vi "Update Controls State.vi"(6 "Controls Need Update In":bool, 7 "Controlst In":refnum<vi>, 8 "Error In (no Error) In":errorcluster, 9 "DigNum Refnum In":refnum<vi>, 10 "Str Refnum In":refnum<vi>, 11 "Display State In":T1={"Show Axes"=FALSE, "Show Y=0"=FALSE, "Controls"={"Type"=enum."Sine", "Periods"=0.0, "Points"=0, "Offset"=0.0, "Amplitdue"=0.0, "Phase"=0.0, "func"=""}, "Show Current Location"=FALSE, "Current Location"=0, "dt"=0.0, "t0"=timestamp(0 s since 1904-01-01), "Format and Units"="%_3p"} caption="State") -> (0 "Error Out":errorcluster, 3 "Display State Out":T1={"Show Axes"=FALSE, "Show Y=0"=FALSE, "Controls"={"Type"=enum."Sine", "Periods"=0.0, "Points"=0, "Offset"=0.0, "Amplitdue"=0.0, "Phase"=0.0, "func"=""}, "Show Current Location"=FALSE, "Current Location"=0, "dt"=0.0, "t0"=timestamp(0 s since 1904-01-01), "Format and Units"="%_3p"} caption="State")   [LabVIEW 2012, in "Waveform Control.xctl"]
doc: "Updates the function generator controls from the state"
uses:
  Waveform Control.xctl
  Controls/Waveform State.ctl
  FP Controls.ctl
  Function Types.ctl
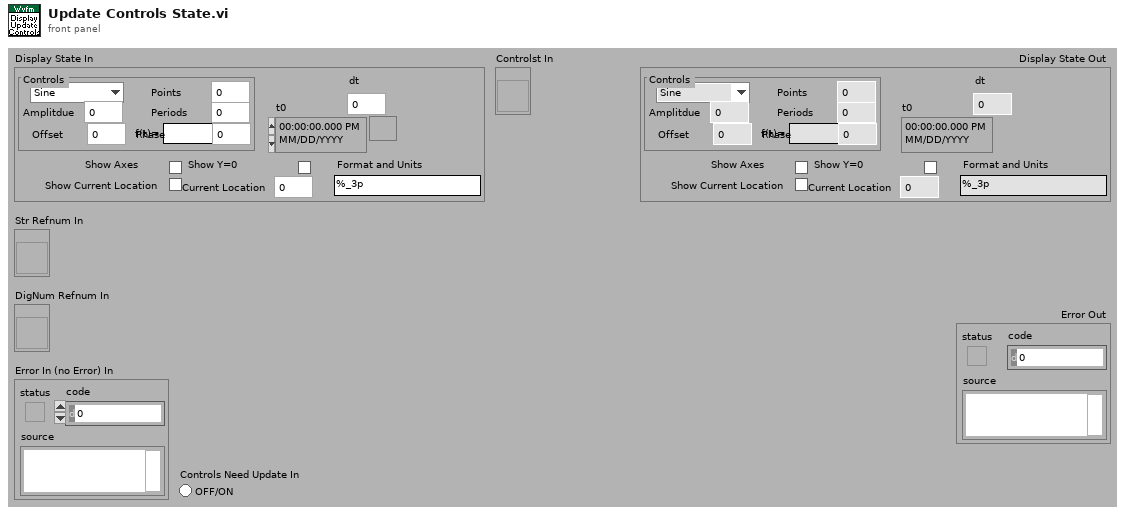
[diagram p1: front panel]
types:
  T1 = typedef "Waveform Control.xctl/Waveform State.ctl" = cluster{"Show Axes":bool, "Show Y=0":bool, "Controls":T2, "Show Current Location":bool, "Current Location":i32, "dt":dbl, "t0":timestamp, "Format and Units":string}
  T2 = typedef "Waveform Control.xctl/FP Controls.ctl" = cluster{"Type":T3, "Periods":dbl, "Points":i32, "Offset":dbl, "Amplitdue":dbl, "Phase":dbl, "func":string}
  T3 = typedef "Waveform Control.xctl/Function Types.ctl" = enum16{"Level", "Sine", "Triangle", "Ramp", "Saw Tooth", "Square", "Function"}
  T4 = cluster{"Type":T3, "Periods":dbl, "Points":i32, "Offset":dbl, "Amplitdue":dbl, "Starting Phase":dbl, "func":string}
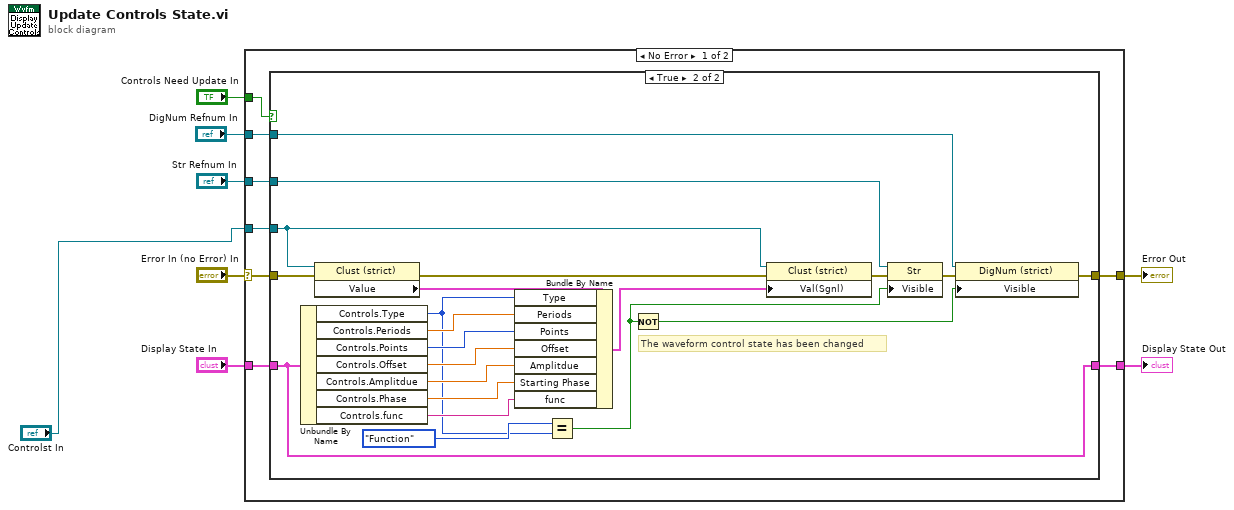
[diagram p0: block diagram]
diagram:
  n1 = case shown="No Error" "Error In (no Error) In" {
    selector: "Error In (no Error) In" -> [w10 w40]
    tunnel: [w16 w40] -> w8
    tunnel: "Display State In" -> [w15 _]
    tunnel: "Controlst In" -> [w14 _]
    tunnel: "Str Refnum In" -> [w13 _]
    tunnel: "DigNum Refnum In" -> [w12 _]
    tunnel: "Controls Need Update In" -> [w9 _]
    tunnel: [w11 _] -> w2
    frame No Error {
      n2 = case shown="True" w9 {
        tunnel: [w17 w39] -> w16
        tunnel: w15 -> [w18 w20]
        tunnel: w14 -> [_ w38]
        tunnel: w13 -> [_ w37]
        tunnel: w12 -> [_ w36]
        tunnel: [w18 w20] -> w11
        tunnel: w10 -> [w17 w19]
        frame False {
        }
        frame True {
          # "The waveform control state has been changed"
          n3 = Unbundle By Name(w20) -> ("Controls.Type"=w21:T3, "Controls.Periods"=w30:dbl, "Controls.Points"=w29:i32, "Controls.Offset"=w28:dbl, "Controls.Amplitdue"=w27:dbl, "Controls.Phase"=w26:dbl, "Controls.func"=w25:string)
          n4 = property on="Property Node" class="Clust (strict)"(reference=w38, error in=w19) -> (error out=w22:errorcluster, "Value"=w31:T4)  [unwired: 1 out]
          n5 = Bundle By Name(cluster=w31, "Type"=w21, "Periods"=w30, "Points"=w29, "Offset"=w28, "Amplitdue"=w27, "Starting Phase"=w26, "func"=w25) -> (w24:T4)
          n6 = Equal?(x=Function_Types."Function" ("Type"), y=w21) -> (x = y?=w34:bool)
          n7 = Not(x=w34) -> (.not. x?=w33:bool)
          n8 = property on="Property Node" class="Clust (strict)"(reference=w38, error in=w22, "Val(Sgnl)"=w24) -> (error out=w23:errorcluster)  [unwired: 1 out]
          n9 = property on="Property Node" class="Str"(reference=w37, error in=w23, "Visible"=w34) -> (error out=w32:errorcluster)  [unwired: 1 out]
          n10 = property on="Property Node" class="DigNum (strict)"(reference=w36, error in=w32, "Visible"=w33) -> (error out=w39:errorcluster)  [unwired: 1 out]
        }
      }
    }
    frame Error {
    }
  }
  "Error Out" <- w8
  "Display State Out" <- w2
